vi "Division.vi"() -> ()   [LabVIEW 2024]
panel:
  out "quotient":dbl
  out "remainder":dbl
  in  "Numeric 2":dbl
  in  "Numeric":dbl
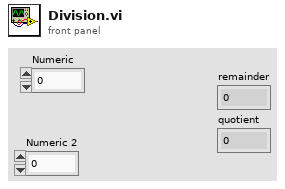
[diagram p1: front panel]
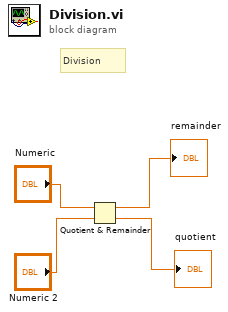
[diagram p0: block diagram]
diagram:
  # "Division"
  n1 = Quotient & Remainder(x="Numeric", y="Numeric 2") -> (x-y*floor(x/y)=→"remainder":dbl, floor(x/y)=→"quotient":dbl)
